vi "Exemplo Atraso.vi"() -> ()   [LabVIEW 2017]
panel:
  out "Mensagem":string
  out "Alerta":bool
  out "Segundos":dbl
  out "Minutos":dbl
  out "Horas":dbl
  in  "Tempo Total em Segundos":dbl
  in  "Stop Button":bool
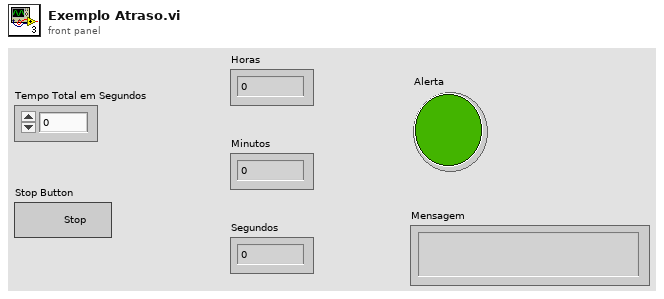
[diagram p1: front panel]
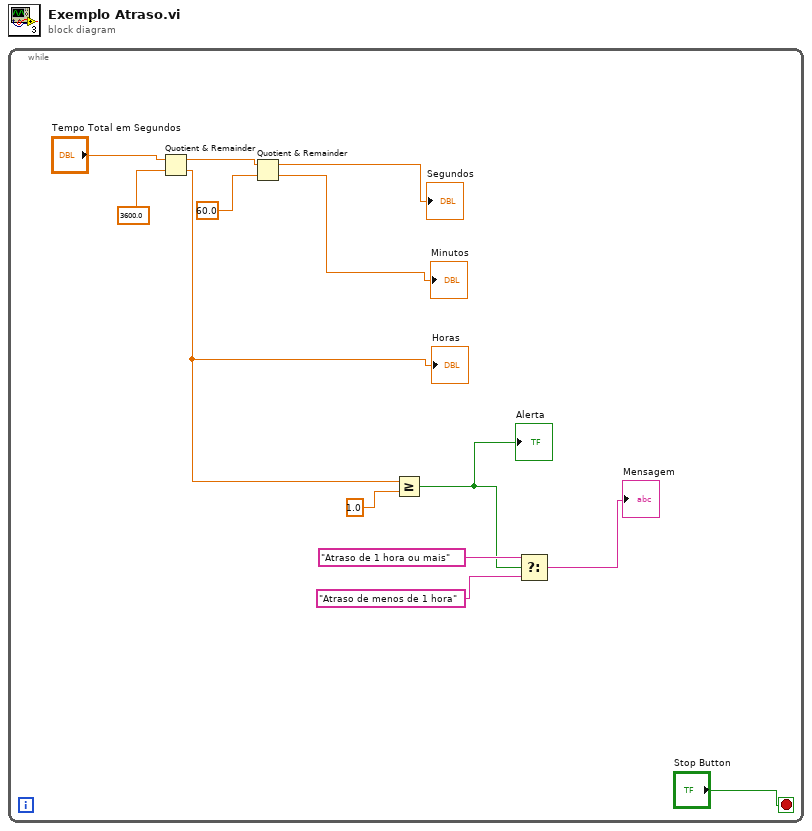
[diagram p0: block diagram]
diagram:
  n1 = while {
    stop <- "Stop Button" stop-if-true
    n2 = Quotient & Remainder(x="Tempo Total em Segundos", y=3600.0) -> (x-y*floor(x/y)=w11:dbl, floor(x/y)=w6:dbl)
    "Horas" <- w6
    n3 = Quotient & Remainder(x=w11, y=60.0) -> (x-y*floor(x/y)=→"Segundos":dbl, floor(x/y)=→"Minutos":dbl)
    n4 = Greater Or Equal?(x=w6, y=1.0) -> (x >= y?=w1:bool)
    "Alerta" <- w1
    n5 = Select(t="Atraso de 1 hora ou mais", s=w1, f="Atraso de menos de 1 hora") -> (s? t:f=→"Mensagem":string)
  }
